vi "position1.vi"() -> ()   [LabVIEW 2023, in "Shared variables.lvlib"]
uses:
  Shared variables.lvlib
panel:
  out "position1":dbl[][](array[numeric])
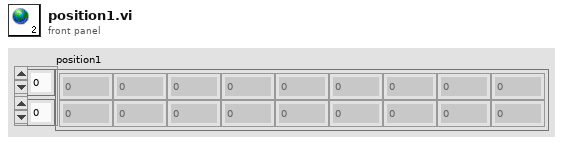
[diagram p1: front panel]
diagram:
